vi "Row_Sum and Col_Sum.vi"(0 "Image_ColorMask":i16[][](array[numeric]), 5 "error in (no error)":errorcluster) -> (14 "Row_Sum":i16[](array[numeric]), 15 "Col_Sum":i16[](array[numeric]), 19 "error out":errorcluster)   [LabVIEW 2013]
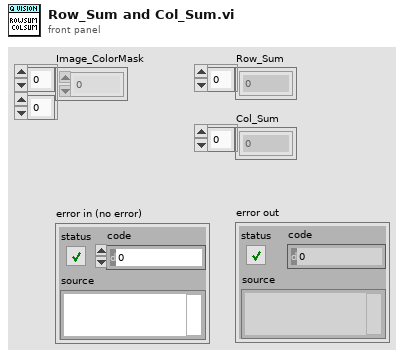
[diagram p1: front panel]
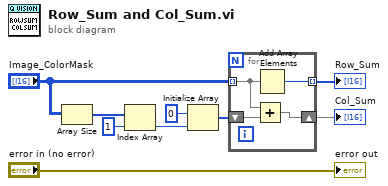
[diagram p0: block diagram]
diagram:
  n1 = Array Size(array="Image_ColorMask") -> (size(s)=w4:i32[])
  n2 = Index Array(array=w4, index=1) -> (element=w6:i32)
  n3 = Initialize Array(i16 0 ("element"), w6) -> (w5:i16[])
  n4 = for {
    tunnel: "Image_ColorMask" -> [w12] mode=indexing
    shift-right: [w11] -> w9
    shift-left: w5 -> [w13]
    tunnel: [w10] -> w8 mode=indexing
    n5 = Add(x=w12, y=w13) -> (x+y=w11:i16[])
    n6 = Add Array Elements(numeric array=w12) -> (sum=w10:i16)
  }
  "Col_Sum" <- w9
  "Row_Sum" <- w8
  "error out" <- "error in (no error)"
